vi "Get Topic Enqueuer.vi"(5 "Channel Class":refnum<class "Pub Sub Message Channel.lvclass">, 7 "Create if not exist? (T)":bool=TRUE, 8 "error in (no error)":errorcluster, 11 "Topic":string) -> (0 "error out":errorcluster, 1 "Topic Enqueuer":refnum<class "Message Enqueuer.lvclass">, 2 "topic not found?":bool, 3 "Channel Out":refnum<class "Pub Sub Message Channel.lvclass">)   [LabVIEW 2020, in "Actor Pub Sub Channels.lvlib"]
uses:
  Actor Pub Sub Channels.lvlib
  <vilib>/ActorFramework/Message Enqueuer/Message Enqueuer.lvclass
  Pub Sub Message Channel/Pub Sub Message Channel.lvclass
  Pub Sub Message Channel/Get Channel Enqueuer.vi
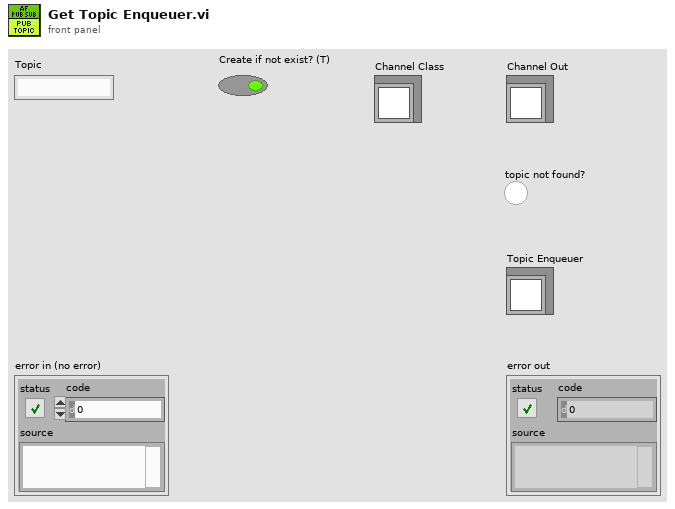
[diagram p1: front panel]
types:
  T1 = enum16{"Nothing", "Get Channel", "Get Or Create Channel", "Close Channel", "Dispose"}
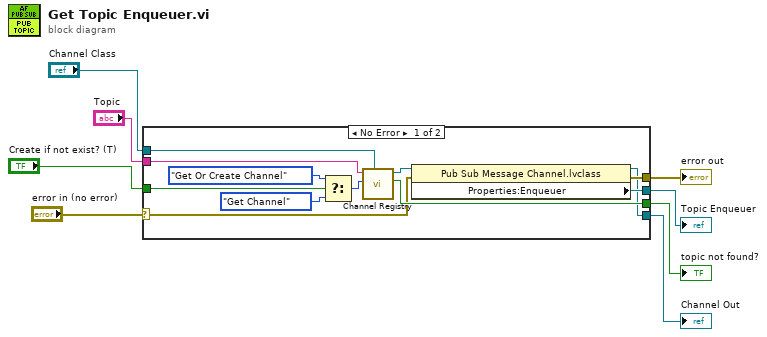
[diagram p0: block diagram]
diagram:
  n1 = case shown="No Error" "error in (no error)" {
    selector: "error in (no error)" -> [w14 w22]
    tunnel: "Create if not exist? (T)" -> [w18 _]
    tunnel: [w16 _] -> w7
    tunnel: "Topic" -> [w15 _]
    tunnel: [w13 w22] -> w4
    tunnel: [w11 _] -> w3
    tunnel: "Channel Class" -> [w10 w21]
    tunnel: [w9 w21] -> w1
    frame No Error {
      n2 = Select(t=T1."Get Or Create Channel" ("Action"), s=w18, f=T1."Get Channel") -> (s? t:f=w19:T1)
      n3 = call "Channel Registry.vi"("New Channel Class"=w10, "Action"=w19, "Topic"=w15) -> ("topic not found?"=w16:bool, "Pub Sub Message Channel"=w12:refnum<class "Pub Sub Message Channel.lvclass">)  [unwired: 6 in, 1 out]
      n4 = property class="Pub Sub Message Channel.lvclass"(reference=w12, error in=w14) -> (reference out=w9:refnum<class "Pub Sub Message Channel.lvclass">, error out=w13:errorcluster, "Properties:Enqueuer"=w11:refnum<class "Message Enqueuer.lvclass">)
    }
    frame Error {
    }
  }
  "topic not found?" <- w7
  "error out" <- w4
  "Topic Enqueuer" <- w3
  "Channel Out" <- w1
